vi "Set Speed Steps.vi"(8 "error in (no error)":errorcluster, 10 "Step ref in":refnum<vi>, 11 "Speed ref in":refnum<vi>) -> (0 "error out":errorcluster)   [LabVIEW 2010, in "SignalWriterMH110203USBStepperMotor.lvclass"]
uses:
  SignalWriterMH110203USBStepperMotor.lvclass
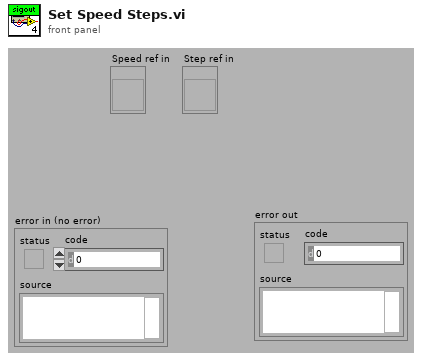
[diagram p1: front panel]
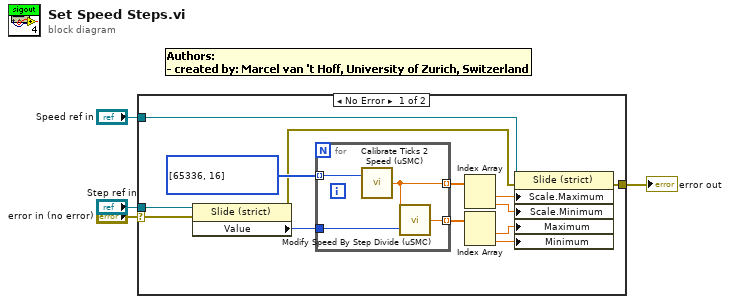
[diagram p0: block diagram]
diagram:
  n1 = case shown="No Error" "error in (no error)" {
    selector: "error in (no error)" -> [w5 w22]
    tunnel: "Step ref in" -> [w17 _]
    tunnel: "Speed ref in" -> [w8 _]
    tunnel: [w6 w22] -> w2
    frame No Error {
      n2 = property class="Slide (strict)"(reference=w17, error in=w5) -> (error out=w7:errorcluster, "Value"=w15:u8)  [unwired: 1 out]
      n3 = for {
        tunnel: u16[] [65336, 16] -> [w21] mode=indexing
        tunnel: w15 -> [w20]
        tunnel: [w19] -> w14 mode=indexing
        tunnel: [w18] -> w13 mode=indexing
        n4 = call "Calibrate Ticks 2 Speed (uSMC).vi"("speed ticks"=w21) -> ("speed value (units)"=w19:dbl)  [unwired: 1 in]
        n5 = call "Modify Speed By Step Divide (uSMC).vi"("Step"=w20, "Speed"=w19) -> ("speed"=w18:dbl)
      }
      n6 = Index Array(array=w14) -> (element #1=w12:dbl, element #2=w11:dbl)  [unwired: 2 in]
      n7 = Index Array(array=w13) -> (element #1=w10:dbl, element #2=w9:dbl)  [unwired: 2 in]
      n8 = property class="Slide (strict)"(reference=w8, error in=w7, "Scale.Maximum"=w12, "Scale.Minimum"=w11, "Maximum"=w10, "Minimum"=w9) -> (error out=w6:errorcluster)  [unwired: 1 out]
    }
    frame Error {
    }
  }
  "error out" <- w2
